vi "MTMount_issueCommand_enableCamWrap.vi"(8 "error in (no error)":errorcluster, 11 "command_enableCamWrap_Ctl":T1) -> (0 "error out":errorcluster, 2 "function return":i32, 3 "command_enableCamWrap_Ctl out":T1)   [LabVIEW 2018, in "SALLV_MTMount.lvlib"]
doc: "int MTMount_shm_issueCommand_enableCamWrapLV(MTMount_command_enableCamWrapLV *command_enableCamWrap_Ctl );"
uses:
  SALLV_MTMount.lvlib
  DataTypes/command_enableCamWrap.ctl
  SALLV_MTMount.so
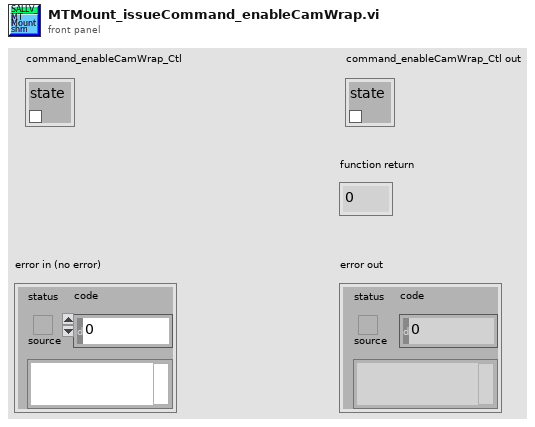
[diagram p1: front panel]
types:
  T1 = typedef "SALLV_MTMount.lvlib/command_enableCamWrap.ctl" = cluster{"state":bool}
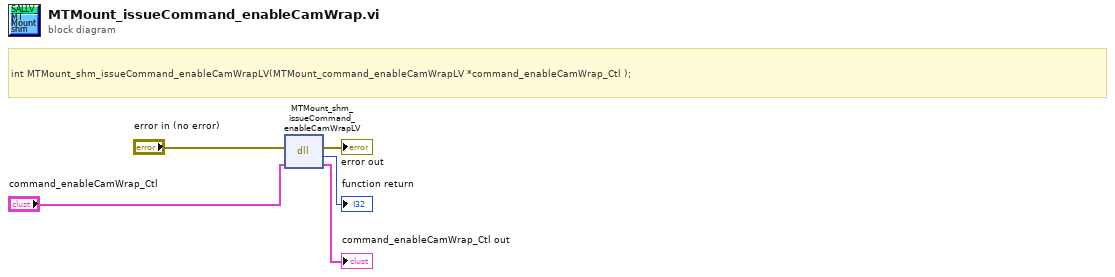
[diagram p0: block diagram]
diagram:
  # "int MTMount_shm_issueCommand_enableCamWrapLV(MTMount_command_enableCamWrapLV *command_enableCamWrap_Ctl );"
  n1 = dll-call lib="home/ttsai/Document/salApiMTMount/SALLV_MTMount/SALLV_MTMount.*" fn="MTMount_shm_issueCommand_enableCamWrapLV"(error in="error in (no error)", "command_enableCamWrap_Ctl"="command_enableCamWrap_Ctl") -> (error out=→"error out":errorcluster, →"function return":i32, "command_enableCamWrap_Ctl"=→"command_enableCamWrap_Ctl out":T1)  [unwired: 2 in, 1 out]
